vi "Do Request.vi"(7 "Processing In":refnum<class "Processing.lvclass">, 11 "SSEHomeController in":refnum<class "SSEHomeController.lvclass">) -> (0 "error out":errorcluster, 5 "Processing":refnum<class "Processing.lvclass">)   [LabVIEW 2020, in "Server Sent Events Example.lvlib" / "SSEHomeController.lvclass"]
doc: "A controller's main job is to respond to a request by generating a response. The response value must be specified by calling Set Response.vi on the Processing class that's passed through the VI otherwise an error will be generated.\n\nThere are several helpers available for common response types:\nGenerating HTML content programmatically - Create Basic Response.vi\nStreaming a file from disk - Create File Response.vi\nRedirecting the user to another URL - Create Redirect Response.vi\n\nFile responses are streamed in chunks and do not load the entire file into memory at once to send in the response which allows serving large files more efficiently."
uses:
  SSEHomeController.lvclass
  lv-http-server/HTTP Server/Processing/Processing.lvclass
  lv-http-server/HTTP Server/Processing/Processing.lvclass/Processing.ctl
  lv-http-util/HTTP Utils/Response/Response.lvclass
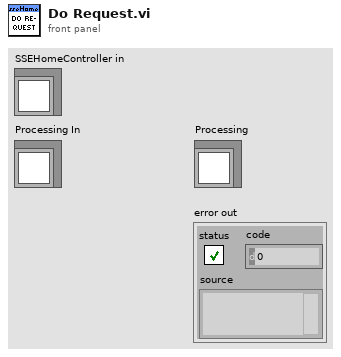
[diagram p1: front panel]
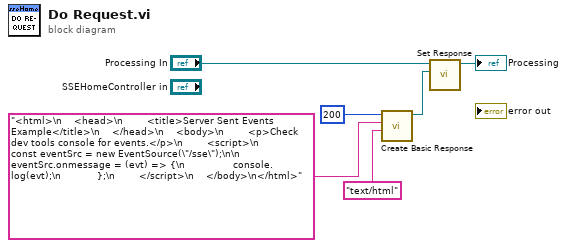
[diagram p0: block diagram]
diagram:
  n1 = call "Create Basic Response.vi"("Content-Type (text/plain)"="text/html", "Payload"="<html>\n    <head>\n        <title>Server Sent Events Example</title>\n    </head>\n    <body>\n        <p>Check dev tools console for events.</p>\n        <script>\n            const eventSrc = new EventSource(\"/sse\");\n\n            eventSrc.onmessage = (evt) => {\n                console.log(evt);\n            };\n        </script>\n    </body>\n</html>", "Status Code"=u16 200) -> ("Response out"=w2:refnum<class "Response.lvclass">)  [unwired: 7 in, 1 out]
  n2 = call "Set Response.vi"("Response"=w2, "Processing in"="Processing In") -> ("Processing out"=→"Processing":refnum<class "Processing.lvclass">)  [unwired: 9 in]
